vi "ff_num_of_device_renames_necessary.vi"(10 "pdTag list":string[](array[string])) -> (2 "num of renames necessary":i32)   [LabVIEW 2012]
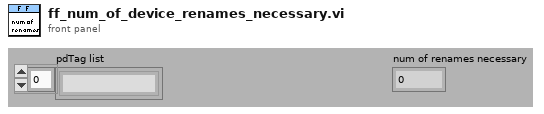
[diagram p1: front panel]
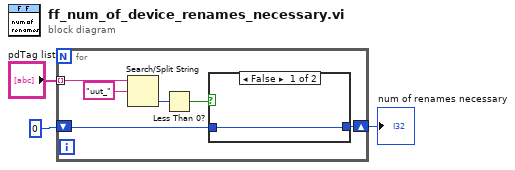
[diagram p0: block diagram]
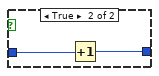
[diagram p2: hidden frame]
diagram:
  n1 = for {
    tunnel: "pdTag list" -> [w9] mode=indexing
    shift-right: [w4] -> w1
    shift-left: 0 -> [w5]
    n2 = Search/Split String(string=w9, search string/char (-)="uut_") -> (offset of match=w7:i32)  [unwired: 1 in, 2 out]
    n3 = Less Than 0?(x=w7) -> (x < 0?=w6:bool)
    n4 = case shown="False" w6 {
      tunnel: w5 -> [w10 w12]
      tunnel: [w10 w11] -> w4
      frame False {
      }
      frame True {
        n5 = Increment(x=w12) -> (x+1=w11:i32)
      }
    }
  }
  "num of renames necessary" <- w1
